vi "Default Settings.vi"(8 "error in (no error)":errorcluster, 11 "Sensor Dispense in":refnum<class "Sensor Dispense.lvclass">) -> (0 "error out":errorcluster, 3 "Sensor Dispense out":refnum<class "Sensor Dispense.lvclass">)   [LabVIEW 2020, in "Sensor Dispense.lvclass"]
uses:
  Projects/Sensor Dispense.lvclass
  Dispense.lvclass
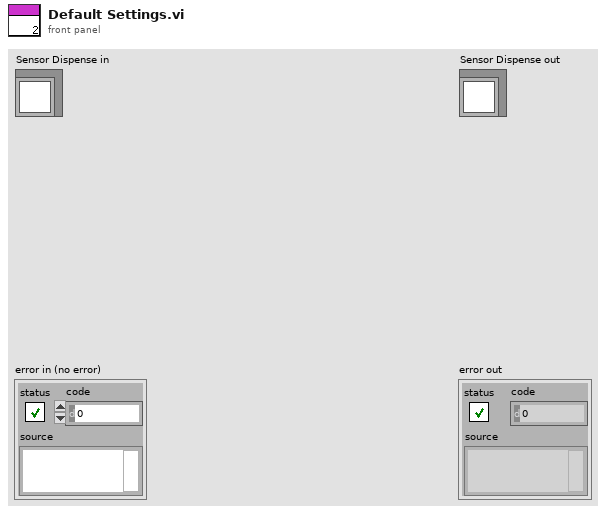
[diagram p1: front panel]
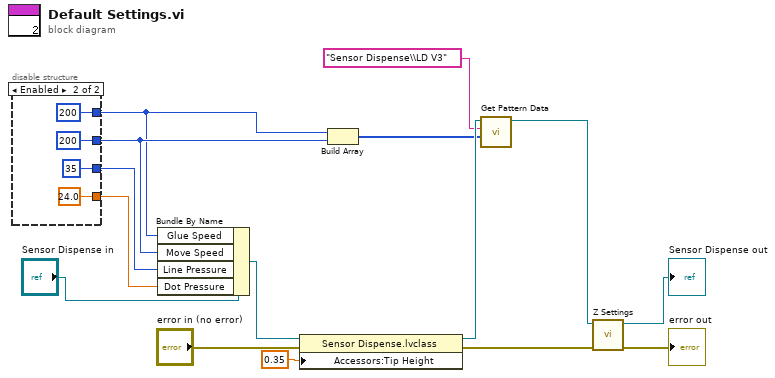
[diagram p0: block diagram]
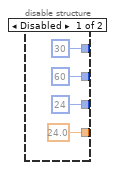
[diagram p2: hidden frame]
diagram:
  n1 = disable-structure shown="Enabled" {
    disable-tunnel: [60 200] -> w4
    disable-tunnel: [30 200] -> w3
    disable-tunnel: [24.0 ("Dot Pressure") 24.0 ("Dot Pressure")] -> w2
    disable-tunnel: [24 35] -> w1
    frame Disabled {
    }
    frame Enabled {
    }
  }
  n2 = Bundle By Name(cluster="Sensor Dispense in", "Glue Speed"=w3, "Move Speed"=w4, "Line Pressure"=w1, "Dot Pressure"=w2) -> (w15:refnum<class "Sensor Dispense.lvclass">)
  n3 = property class="Sensor Dispense.lvclass"(reference=w15, error in="error in (no error)", "Accessors:Tip Height"=0.35) -> (reference out=w12:refnum<class "Sensor Dispense.lvclass">, error out=w6:errorcluster)
  n4 = Build Array(w3, w4) -> (w10:i32[])
  n5 = call "Get Pattern Data.vi"("File Name"=w10, "Folder Name"="Sensor Dispense\\LD V3", "Dispense.lvclass"=w12) -> ("Dispense Out"=w9:refnum<class "Sensor Dispense.lvclass">)  [unwired: 8 in]
  n6 = call-dynamic "Z Settings.vi"("error in (no error)"=w6, "Dispense in"=w9) -> ("error out"=→"error out":errorcluster, "Dispense out"=→"Sensor Dispense out":refnum<class "Sensor Dispense.lvclass">)  [unwired: 8 in]
